vi "Write States.vi"(8 "error in (no error)":errorcluster, 10 "States":T1, 11 "AttackerStopTactic in":refnum<class "AttackerStopTactic.lvclass">) -> (0 "error out":errorcluster, 3 "AttackerStopTactic out":refnum<class "AttackerStopTactic.lvclass">)   [LabVIEW 2023, in "AttackerStopTactic.lvclass"]
uses:
  AttackerStopTactic.lvclass
  States.ctl
  AttackerStopTactic.lvclass/AttackerStopTactic.ctl
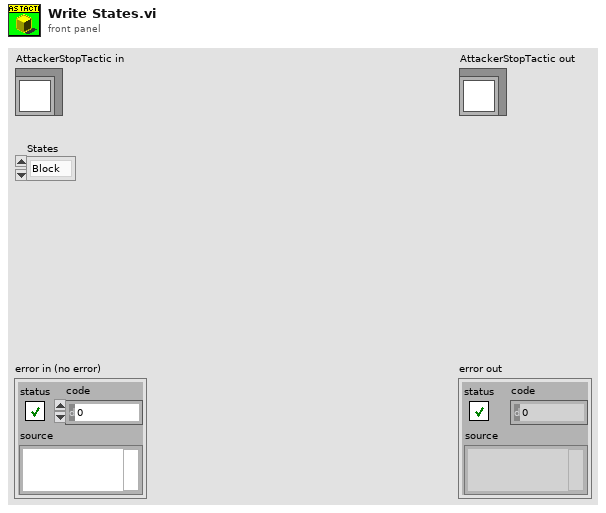
[diagram p1: front panel]
types:
  T1 = typedef "AttackerStopTactic.lvclass/States.ctl" = enum16{"Block", "AimGoal", "Exit"}
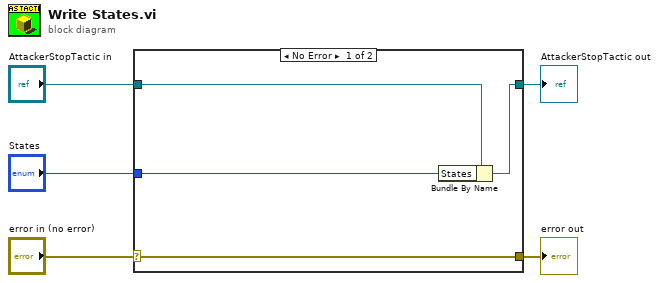
[diagram p0: block diagram]
diagram:
  n1 = case shown="No Error" "error in (no error)" {
    selector: "error in (no error)" -> [w9 w10]
    tunnel: [w9 w10] -> w4
    tunnel: [w7 w11] -> w2
    tunnel: "AttackerStopTactic in" -> [w8 w11]
    tunnel: "States" -> [w6 _]
    frame No Error {
      n2 = Bundle By Name(cluster=w8, "States"=w6) -> (w7:refnum<class "AttackerStopTactic.lvclass">)
    }
    frame Error {
    }
  }
  "error out" <- w4
  "AttackerStopTactic out" <- w2
